vi "Boil off rates.vi"() -> ()   [LabVIEW 2015]
panel:
  out "x+y":dbl
  out "Array":dbl[](array[numeric]) format="%.3g"
  out "time (S)":dbl
  in  "file path out":path
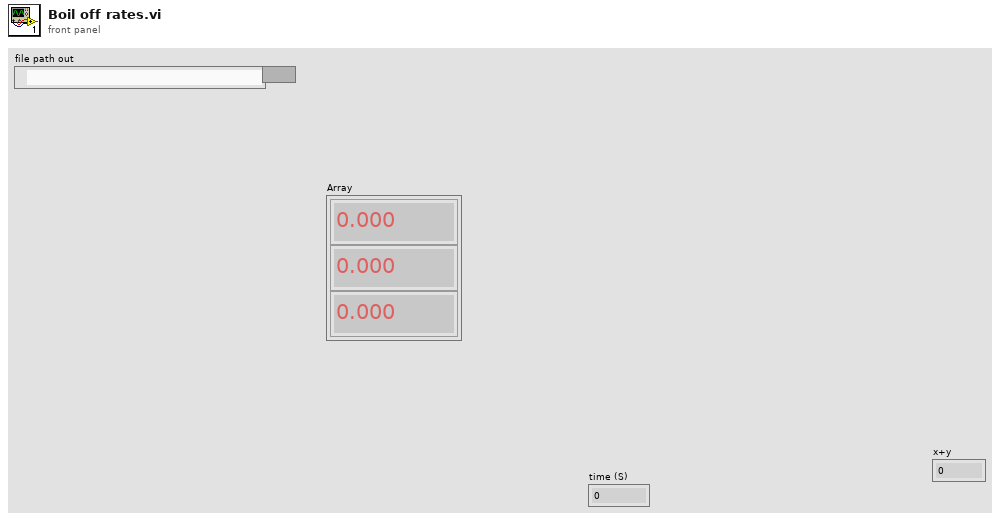
[diagram p1: front panel]
types:
  T1 = enum16{"open", "open or create", "create or replace", "create", "open (read-only)"}
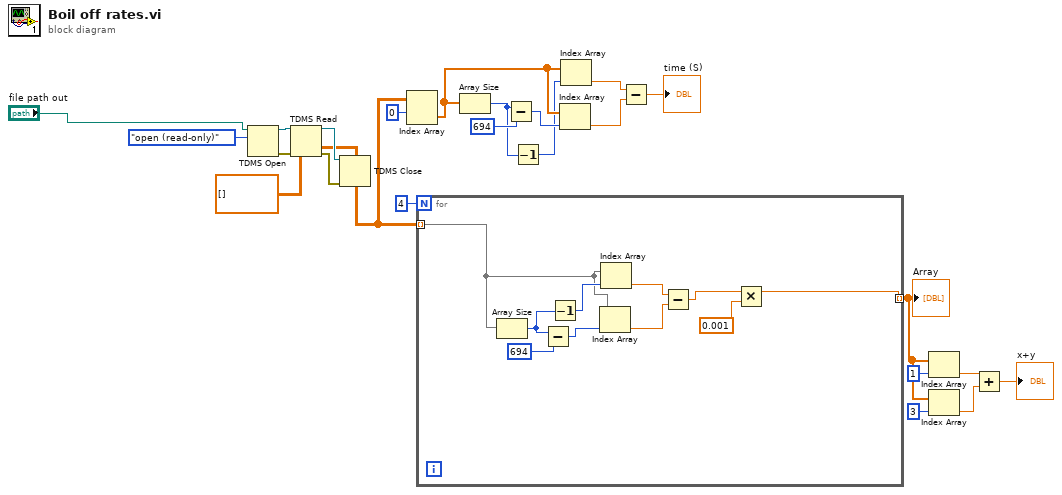
[diagram p0: block diagram]
diagram:
  n1 = TDMS Open(10:T1."open (read-only)" ("operation (0:open)"), 11:"file path out") -> (0:w21:errorcluster, 3:w22:refnum<k34>)  [unwired: 5 in]
  n2 = TDMS Read(0:w22, 11:w21, 12:dbl[][] []) -> (4:w18:refnum<k34>, 10:w16:dbl[][], 15:w19:errorcluster)  [unwired: 5 in, 3 out]
  n3 = TDMS Close(8:w19, 11:w18) -> ()  [unwired: 2 out]
  n4 = Index Array(array=w16, index (row)=0) -> (element=w14:dbl[])  [unwired: 1 in]
  n5 = for {
    N: 4 -> [_]
    tunnel: w16 -> [w26] mode=indexing
    tunnel: [w25] -> w6 mode=indexing
    n6 = Array Size(array=w26) -> (size(s)=w33:i32)
    n7 = Subtract(x=w33, y=694) -> (x-y=w28:i32)
    n8 = Decrement(x=w33) -> (x-1=w29:i32)
    n9 = Index Array(array=w26, index=w28) -> (element=w31:dbl)
    n10 = Index Array(array=w26, index=w29) -> (element=w32:dbl)
    n11 = Subtract(x=w32, y=w31) -> (x-y=w30:dbl)
    n12 = Multiply(x=w30, y=0.001) -> (x*y=w25:dbl)
  }
  "Array" <- w6
  n13 = Array Size(array=w14) -> (size(s)=w10:i32)
  n14 = Subtract(x=w10, y=694) -> (x-y=w9:i32)
  n15 = Decrement(x=w10) -> (x-1=w8:i32)
  n16 = Index Array(array=w14, index=w9) -> (element=w12:dbl)
  n17 = Index Array(array=w14, index=w8) -> (element=w13:dbl)
  n18 = Subtract(x=w13, y=w12) -> (x-y=→"time (S)":dbl)
  n19 = Index Array(array=w6, index=1) -> (element=w3:dbl)
  n20 = Index Array(array=w6, index=3) -> (element=w2:dbl)
  n21 = Add(x=w3, y=w2) -> (x+y=→"x+y":dbl)
